vi "receive_data.vi"(5 "error in (no error)":errorcluster) -> (4 "timeout?":bool, 6 "error out":errorcluster)   [LabVIEW 2016, in "BT-Android_interface.lvlib"]
uses:
  BT-Android_interface.lvlib
  mode.ctl
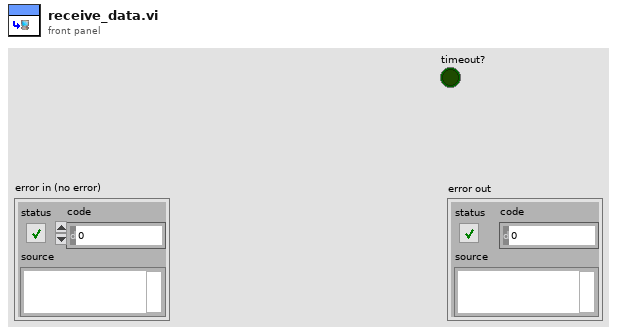
[diagram p1: front panel]
types:
  T1 = typedef "BT-Android_interface.lvlib/mode.ctl" = enum16{"init", "broadcast_data", "receive_data", "close"}
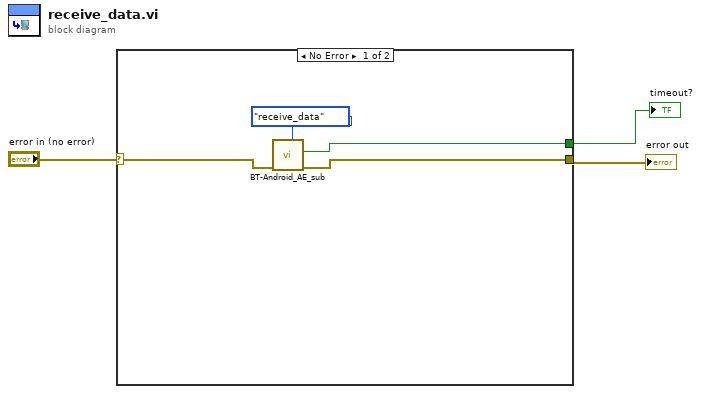
[diagram p0: block diagram]
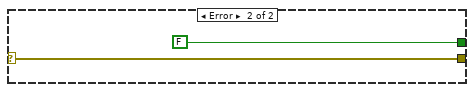
[diagram p2: hidden frame]
diagram:
  n1 = case shown="No Error" "error in (no error)" {
    selector: "error in (no error)" -> [w7 w9]
    tunnel: [w6 w9] -> w2
    tunnel: [w5 FALSE ("timeout?")] -> w1
    frame No Error {
      n2 = call "BT-Android_AE_sub.vi"("mode"=mode."receive_data", "error in (no error)"=w7) -> ("error IO"=w6:errorcluster, "timeout?"=w5:bool)  [unwired: 8 in]
    }
    frame Error {
    }
  }
  "error out" <- w2
  "timeout?" <- w1
